vi "InfiniiVision Get Waveform.vi"(0 "VISA Resource Name":refnum<visa-resource-name>="USB0::0x0957::0x1754::MY48260178::INSTR") -> (4 "error out":errorcluster, 11 "Waveform Data":waveform(dbl)(graph))   [LabVIEW 2018]
uses:
  <vilib>/Waveform/WDTFileIO.llb/Export Waveform To Spreadsheet File.vi
panel:
  in  "# Points (Stop/Single required for >1k)":u16(ring)=3 items=["8M (Single required)", "4M", "2M", "1M", "500k", "200k", "100k", "50k", "20k", "10k", "5k", "2k", "1k", "500", "250", "100"]
  out "# Points":i32
  in  "Timeout Value (ms)":u32=2000
  in  "Create CSV Output File":bool
  in  "Output File":path
  in  "Source":u16(ring) items=["Channel 1", "Channel 2", "Channel 3", "Channel 4", "Math"]
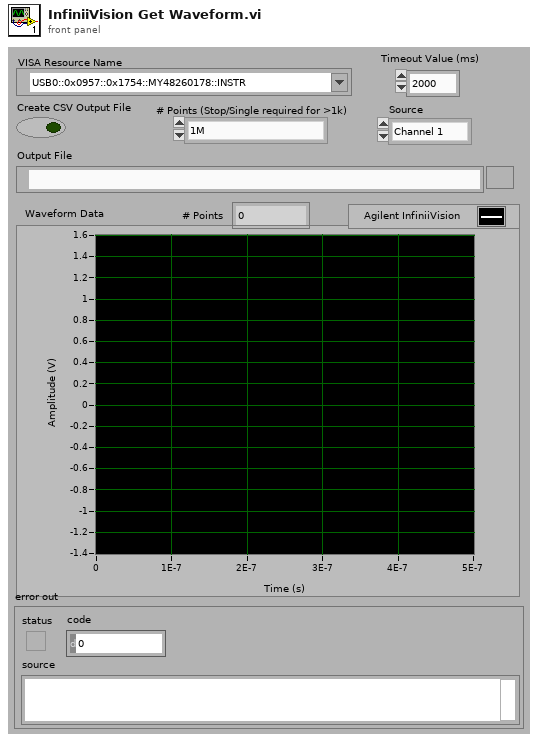
[diagram p1: front panel]
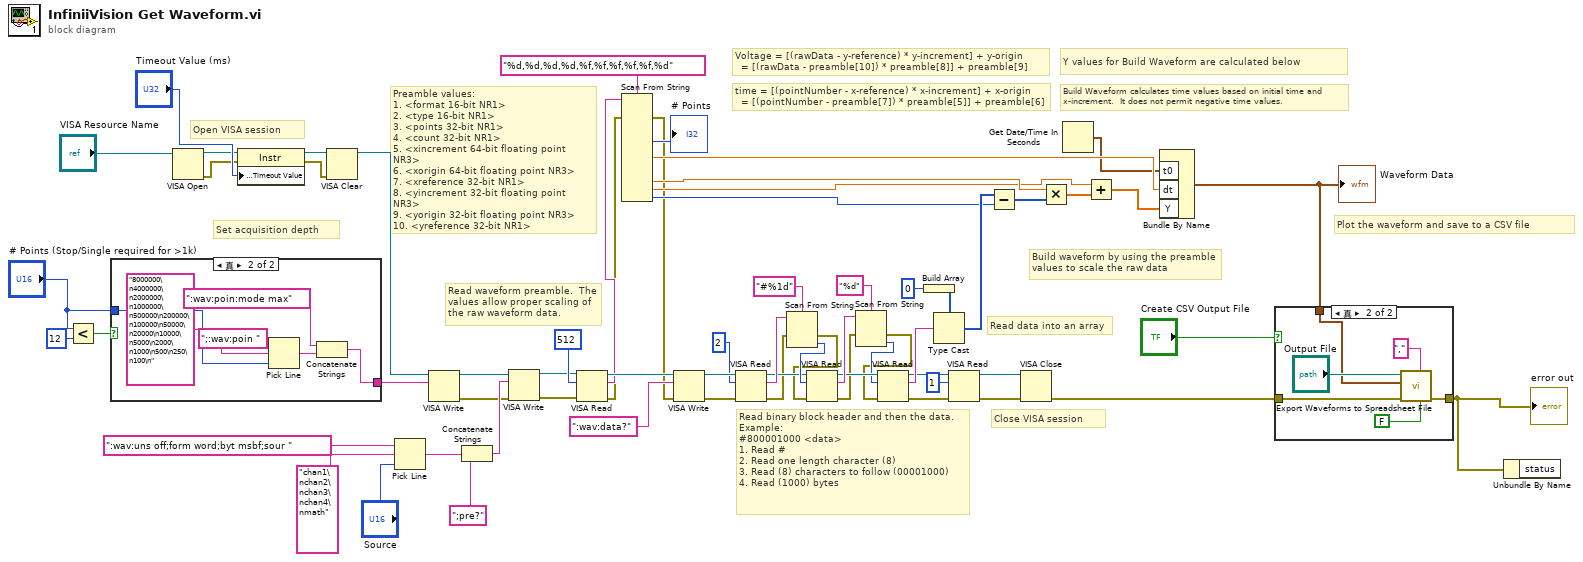
[diagram p0: block diagram]
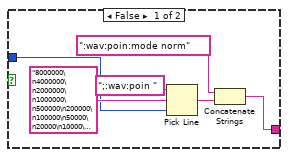
[diagram p2: hidden frame]
diagram:
  # "Close VISA session"
  # "Open VISA session"
  # "Set acquisition depth"
  # "Plot the waveform and save to a CSV file"
  # "Build Waveform calculates time values based on initial time and x-increment.  It does not permit negative time values."
  # "Y values for Build Waveform are calculated below"
  # "Build waveform by using the preamble values to scale the raw data"
  # "Read data into an array"
  # "Read binary block header and then the data.  Example: \n#800001000 <data>\n1. Read #\n2. Read one length character (8)\n3. Read (8) characters to follow (00001000)\n4. Read (1000) bytes"
  # "Read waveform preamble.  The values allow proper scaling of the raw waveform data."
  # "time = [(pointNumber - x-reference) * x-increment] + x-origin\n\t = [(pointNumber - preamble[7]) * preamble[5]] + preamble[6]"
  # "Voltage = [(rawData - y-reference) * y-increment] + y-origin\n\t\t= [(rawData - preamble[10]) * preamble[8]] + preamble[9]"
  # "Preamble values: \n1. <format 16-bit NR1>\n2. <type 16-bit NR1>\n3. <points 32-bit NR1>\n4. <count 32-bit NR1>\n5. <xincrement 64-bit floating point NR3>\n6. <xorigin 64-bit floating point NR3>\n7. <xreference 32-bit NR1>\n8. <yincrement 32-bit floating point NR3>\n9. <yorigin 32-bit floating point NR3>\n10. <yreference 32-bit NR1>"
  n1 = Less?(x="# Points (Stop/Single required for >1k)", y=u16 12) -> (x < y?=w9:bool)
  n2 = case shown="真" w9 {
    tunnel: [w68 w72] -> w14
    tunnel: "# Points (Stop/Single required for >1k)" -> [w69 w73]
    frame False {
      n3 = Pick Line(string ("")=";:wav:poin ", multi-line string="8000000\n4000000\n2000000\n1000000\n500000\n200000\n100000\n50000\n20000\n10000\n5000\n2000\n1000\n500\n250\n100\n", line index=w69) -> (output string=w67:string)
      n4 = Concatenate Strings(":wav:poin:mode norm" ("string"), w67) -> (w68:string)
    }
    frame True {
      n5 = Pick Line(string ("")=";:wav:poin ", multi-line string="8000000\n4000000\n2000000\n1000000\n500000\n200000\n100000\n50000\n20000\n10000\n5000\n2000\n1000\n500\n250\n100\n", line index=w73) -> (output string=w76:string)
      n6 = Concatenate Strings(":wav:poin:mode max" ("string"), w76) -> (w72:string)
    }
  }
  n7 = VISA Open(VISA resource name="VISA Resource Name") -> (VISA resource name=w19:refnum<visa-resource-name>, error out=w18:errorcluster)  [unwired: 4 in]
  n8 = property class="Instr"(reference=w19, error in=w18, "General Settings:Timeout Value"="Timeout Value (ms)") -> (reference out=w17:refnum<visa-resource-name>, error out=w16:errorcluster)
  n9 = VISA Clear(VISA resource name=w17, error in (no error)=w16) -> (VISA resource name out=w13:refnum<visa-resource-name>)  [unwired: 1 out]
  n10 = Pick Line(string ("")=":wav:uns off;form word;byt msbf;sour ", multi-line string="chan1\nchan2\nchan3\nchan4\nmath", line index="Source") -> (output string=w61:string)
  n11 = VISA Write(VISA resource name=w13, write buffer=w14) -> (VISA resource name out=w12:refnum<visa-resource-name>, error out=w11:errorcluster)  [unwired: 1 in, 1 out]
  n12 = Concatenate Strings(w61, ";pre?" ("string")) -> (w62:string)
  n13 = VISA Write(VISA resource name=w12, write buffer=w62, error in (no error)=w11) -> (VISA resource name out=w58:refnum<visa-resource-name>, error out=w57:errorcluster)  [unwired: 1 out]
  n14 = VISA Read(VISA resource name=w58, byte count=u32 512, error in (no error)=w57) -> (VISA resource name out=w56:refnum<visa-resource-name>, read buffer=w31:string, error out=w7:errorcluster)  [unwired: 1 out]
  n15 = Scan From String(format string="%d,%d,%d,%d,%f,%f,%f,%f,%f,%d", input string=w31, error in=w7) -> (error out=w6:errorcluster, output 3=→"# Points":i32, output 5=w24:dbl, output 8=w36:dbl, output 9=w34:dbl, output 10=w29:i32)  [unwired: 16 in, 2 out]
  n16 = VISA Write(VISA resource name=w56, write buffer=":wav:data?", error in (no error)=w6) -> (VISA resource name out=w54:refnum<visa-resource-name>, error out=w53:errorcluster)  [unwired: 1 out]
  n17 = VISA Read(VISA resource name=w54, byte count=u32 2, error in (no error)=w53) -> (VISA resource name out=w48:refnum<visa-resource-name>, read buffer=w51:string, error out=w5:errorcluster)  [unwired: 1 out]
  n18 = Scan From String(format string="#%1d", input string=w51, error in=w5) -> (error out=w4:errorcluster, output 1=w49:i32)  [unwired: 2 in, 2 out]
  n19 = VISA Read(VISA resource name=w48, byte count=w49, error in (no error)=w4) -> (VISA resource name out=w45:refnum<visa-resource-name>, read buffer=w47:string, error out=w3:errorcluster)  [unwired: 1 out]
  n20 = Scan From String(format string="%d", input string=w47, error in=w3) -> (error out=w2:errorcluster, output 1=w44:i32)  [unwired: 2 in, 2 out]
  n21 = VISA Read(VISA resource name=w45, byte count=w44, error in (no error)=w2) -> (VISA resource name out=w40:refnum<visa-resource-name>, read buffer=w41:string, error out=w39:errorcluster)  [unwired: 1 out]
  n22 = Build Array(i16 0 ("element")) -> (w42:i16[])
  n23 = Type Cast(type=w42, x=w41) -> (*(type *) &x=w30:i16[])
  n24 = VISA Read(VISA resource name=w40, byte count=u32 1, error in (no error)=w39) -> (VISA resource name out=w33:refnum<visa-resource-name>, error out=w32:errorcluster)  [unwired: 2 out]
  n25 = Subtract(x=w30, y=w29) -> (x-y=w37:i32[])
  n26 = VISA Close(VISA resource name=w33, error in (no error)=w32) -> (error out=w25:errorcluster)
  n27 = Multiply(x=w36, y=w37) -> (x*y=w35:dbl[])
  n28 = Get Date/Time In Seconds() -> (seconds since 1Jan1904=w23:timestamp)
  n29 = Add(x=w34, y=w35) -> (x+y=w28:dbl[])
  n30 = Bundle By Name("t0"=w23, "dt"=w24, "Y"=w28) -> (w22:waveform(dbl))  [unwired: 1 in]
  "Waveform Data" <- w22
  n31 = case shown="真" "Create CSV Output File" {
    tunnel: w22 -> [_ w82]
    tunnel: w25 -> [w78 w81]
    tunnel: [w78 w79] -> w1
    frame False {
    }
    frame True {
      n32 = call-poly <vilib>:"Export Waveforms to Spreadsheet File.vi"("header? (write header:T)"=FALSE, "delimiter (Tab)"=",", "error in (no error)"=w81, "waveform"=w82, "file path (dialog if empty)"="Output File") -> ("error out"=w79:errorcluster)  [unwired: 5 in, 1 out]
    }
  }
  "error out" <- w1
  n33 = Unbundle By Name(w1) -> ()  [unwired: 1 out]
